vi "getConfiguration.vi"(8 "error in (no error)":errorcluster, 11 "Camera in":refnum<class "Camera.lvclass">) -> (0 "error out":errorcluster, 2 "configuration":T2={"exposure_time_s"=nan, "delay_time_s"=nan, "roi"={"x0"=18446744073709551615, "y0"=18446744073709551615, "x1"=18446744073709551615, "y1"=18446744073709551615}, "timestamp_mode"=65535, "pixelrate"=4294967295, "conversion_factor"=0.0, "trigger_mode"=65535, "acquire_mode"=65535, "acquire_sequence_number"=65535, "metadata_mode"=65535, "noisefilter_mode"=65535, "pixel_format"=0, "binning"={"vert"=0, "horz"=0, "mode"=0}, "auto_exposure"={"region"=0, "min_exposure_s"=0.001, "max_exposure_s"=0.1}} {"conversion_factor" format="%.2g"; "acquire_sequence_number" items=["Undefined"=65535, "OFF"=0, "ON"=1]; "auto_exposure"."region" items=["balanced", "center_based", "corner_based", "full", "custom"]; "binning"."mode" items=["sum", "average"]; "noisefilter_mode" items=["Undefined"=65535, "OFF"=0, "ON"=1]; "exposure_time_s" format="%#_6f"; "timestamp_mode" items=["Undefined"=65535, "OFF"=0, "Binary"=1, "Binary+ASCII"=2, "ASCII"=3]; "acquire_mode" items=["Undefined"=65535, "auto"=0, "external"=1, "external modulate"=2]; "trigger_mode" items=["Undefined"=65535, "auto sequence"=0, "software trigger"=1, "external exposure start & software trigger"=2, "external exposure control"=3, "external synchronized"=4, "fast external exposure control"=5, "external CDS control"=6, "slow external exposure control"=7, "external synchronized HDSDI"=258]; "metadata_mode" items=["Undefined"=65535, "OFF"=0, "ON"=1]}, 3 "Camera out":refnum<class "Camera.lvclass">)   [LabVIEW 2019, in "Camera.lvclass"]
doc: "Gets the current configuration from the camera."
uses:
  Camera.lvclass
  Camera.lvclass/Camera.ctl
  pco.sdk/TimingControl/TimingControl.lvlib
  pco.sdk/ImageSensor/ImageSensor.lvlib
  pco.sdk/RecordingControl/RecordingControl.lvlib
  Controls/binning.ctl
  pco.sdk/GeneralCameraControl/GeneralCameraControl.lvlib
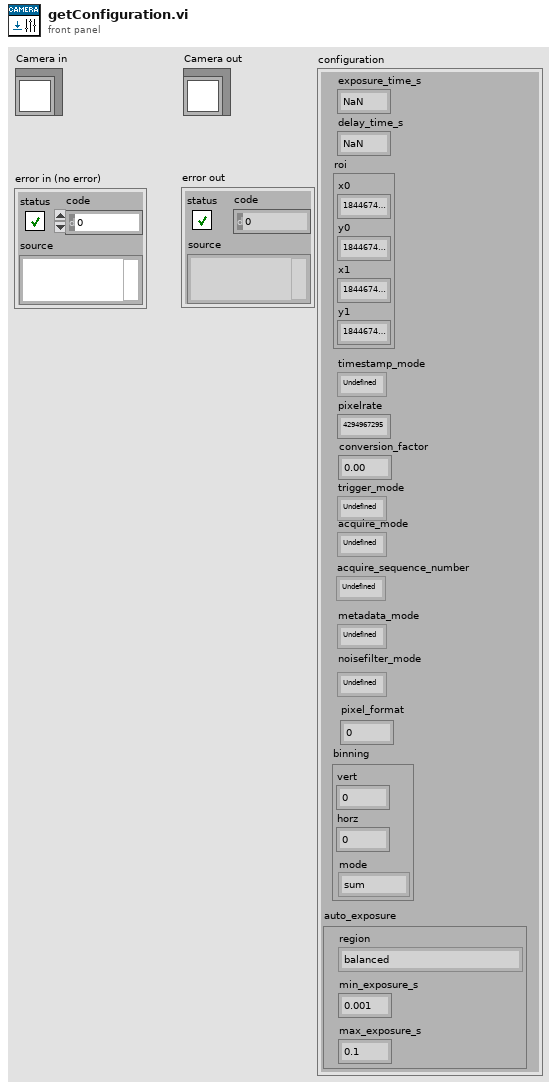
[diagram p1: front panel]
types:
  T1 = typedef "Camera.lvclass/binning.ctl" = cluster{"vert":u16, "horz":u16, "mode":u16}
  T2 = cluster{"exposure_time_s":dbl, "delay_time_s":dbl, "roi":cluster{"x0":u64, "y0":u64, "x1":u64, "y1":u64}, "timestamp_mode":u16, "pixelrate":u32, "conversion_factor":sgl, "trigger_mode":u16, "acquire_mode":u16, "acquire_sequence_number":u32, "metadata_mode":u16, "noisefilter_mode":u16, "pixel_format":u32, "binning":T1, "auto_exposure":cluster{"region":u16, "min_exposure_s":dbl, "max_exposure_s":dbl}}
  T3 = enum16{"SETUP_TYPE_SHUTTERMODE", "SETUP_TYPE_PIXELFORMAT", "SETUP_TYPE_SENSOR_DYNRES"}
  T4 = cluster{"wSensorTypeDESC":u16, "wSensorSubTypeDESC":u16, "wMaxHorzResStdDESC":u16, "wMaxVertResStdDESC":u16, "wMaxHorzResExtDESC":u16, "wMaxVertResExtDESC":u16, "wDynResDESC":u16, "wMaxBinHorzDESC":u16, "wBinHorzSteppingDESC":u16, "wMaxBinVertDESC":u16, "wBinVertSteppingDESC":u16, "wRoiHorStepsDESC":u16, "wRoiVertStepsDESC":u16, "wNumADCsDESC":u16, "wMinSizeHorzDESC":u16, "dwPixelRateDESC":u32[], "wConvFactDESC":u16[], "sCoolingSetpoints":i16[], "wSoftRoiHorStepsDESC":u16, "wSoftRoiVertStepsDESC":u16, "wIRDESC":u16, "wMinSizeVertDESC":u16, "dwMinDelayDESC":u32, "dwMaxDelayDESC":u32, "dwMinDelayStepDESC":u32, "dwMinExposureDESC":u32, "dwMaxExposureDESC":u32, "dwMinExposureStepDESC":u32, "dwMinDelayIRDESC":u32, "dwMaxDelayIRDESC":u32, "dwMinExposureIRDESC":u32, "dwMaxExposureIRDESC":u32, "wTimeTableDESC":u16, "wDoubleImageDESC":u16, "sMinCoolSetDESC":i16, "sMaxCoolSetDESC":i16, "sDefaultCoolSetDESC":i16, "wPowerDownModeDESC":u16, "wOffsetRegulationDESC":u16, "wColorPatternDESC":u16, "wPatternTypeDESC":u16, "wNumCoolingSetpoints":u16, "dwGeneralCapsDESC1":u32, "dwGeneralCapsDESC2":u32, "dwExtSyncFrequency":u32[], "dwGeneralCapsDESC3":u32, "dwGeneralCapsDESC4":u32}
  T5 = cluster{"region":u16, "min_exposure_s":dbl, "max_exposure_s":dbl}
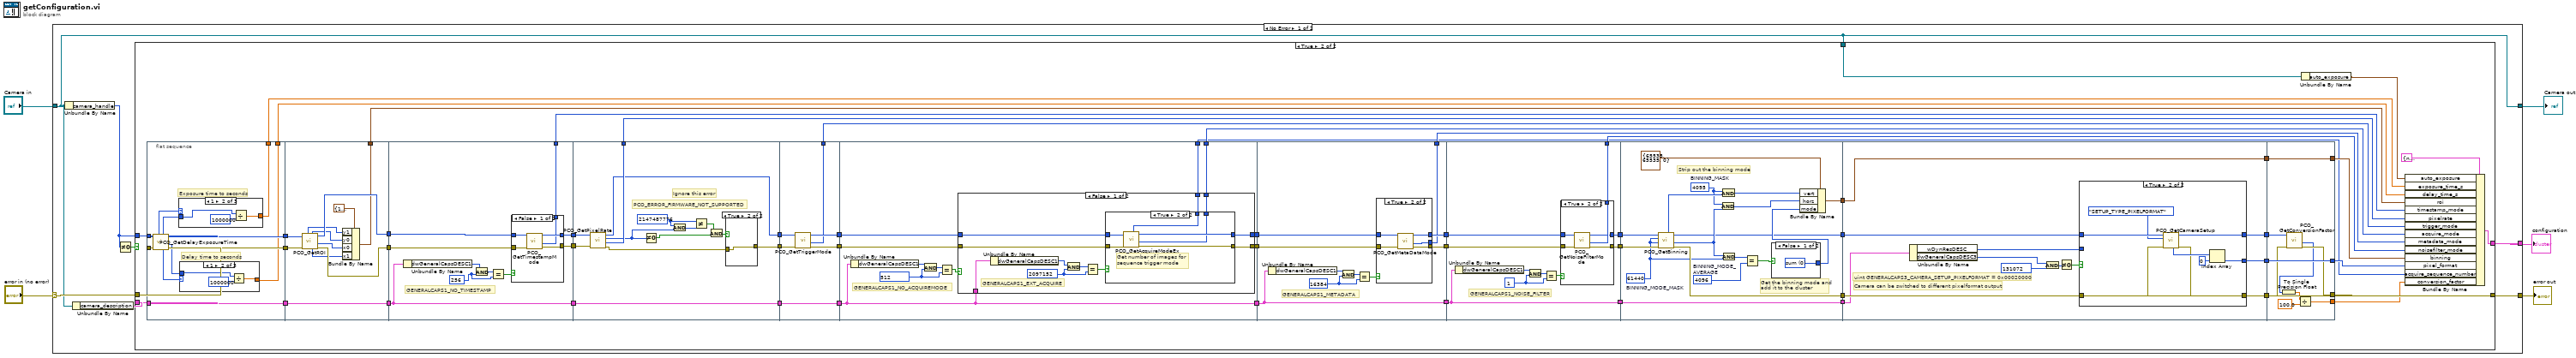
[diagram p0: block diagram]
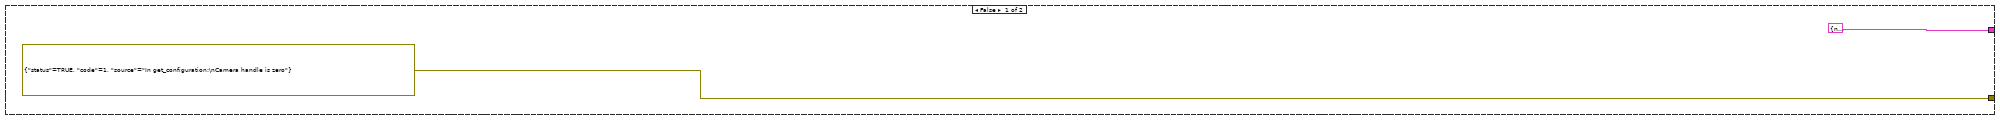
[diagram p2: hidden frame]
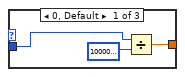
[diagram p3: hidden frame]
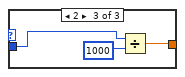
[diagram p4: hidden frame]
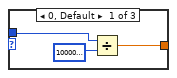
[diagram p5: hidden frame]
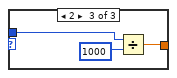
[diagram p6: hidden frame]
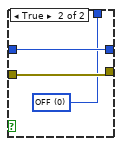
[diagram p7: hidden frame]
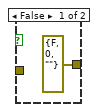
[diagram p8: hidden frame]
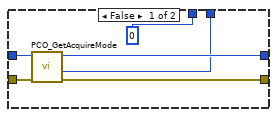
[diagram p9: hidden frame]
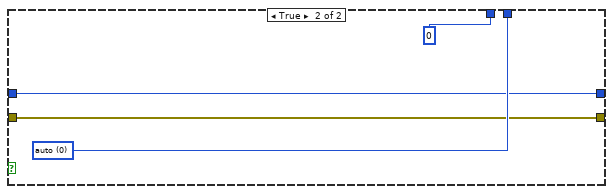
[diagram p10: hidden frame]
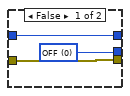
[diagram p11: hidden frame]
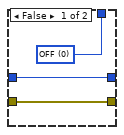
[diagram p12: hidden frame]
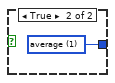
[diagram p13: hidden frame]
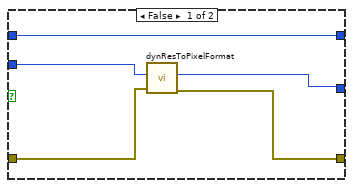
[diagram p14: hidden frame]
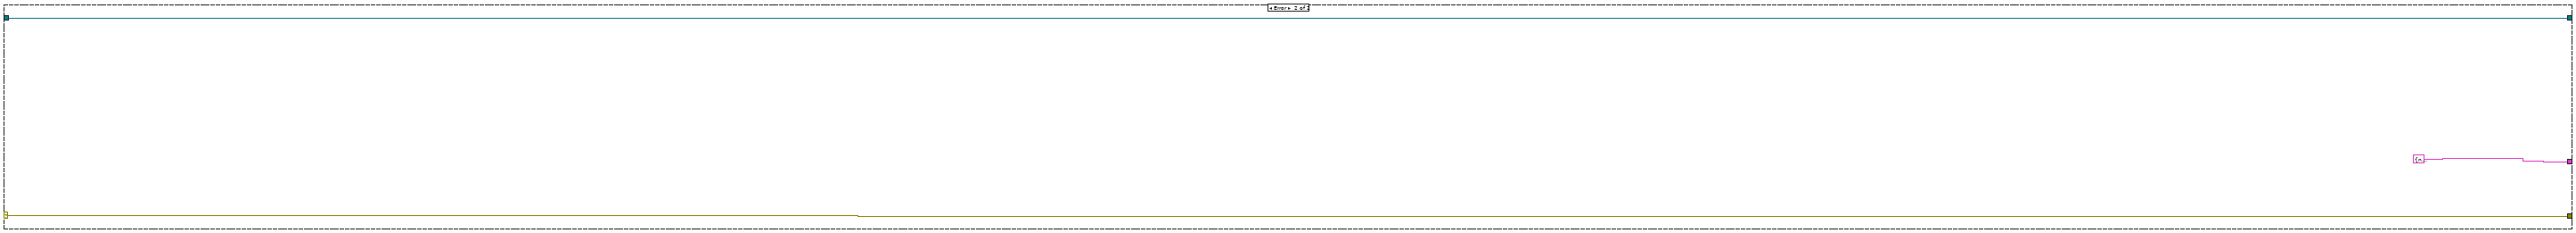
[diagram p15: hidden frame]
diagram:
  n1 = case shown="No Error" "error in (no error)" {
    selector: "error in (no error)" -> [w9 w276]
    tunnel: [w11 w276] -> w4
    tunnel: [w6 w275] -> w2
    tunnel: "Camera in" -> [w6 w275]
    tunnel: [w8 T2 {"exposure_time_s"=nan, "delay_time_s"=nan, "roi"={"x0"=18446744073709551615, "y0"=18446744073709551615, "x1"=18446744073709551615, "y1"=18446744073709551615}, "timestamp_mode"=65535, "pixelrate"=4294967295, "conversion_factor"=0.0, "trigger_mode"=65535, "acquire_mode"=65535, "acquire_sequence_number"=65535, "metadata_mode"=65535, "noisefilter_mode"=65535, "pixel_format"=0, "binning"={"vert"=0, "horz"=0, "mode"=0}, "auto_exposure"={"region"=0, "min_exposure_s"=0.001, "max_exposure_s"=0.1}} ("configuration")] -> w1
    frame No Error {
      n2 = Unbundle By Name(w6) -> ("camera_handle"=w10:u64)
      n3 = Unbundle By Name(w6) -> ("camera_description"=w7:T4)
      n4 = Not Equal To 0?(x=w10) -> (x != 0?=w12:bool)
      n5 = case shown="True" w12 {
        tunnel: [errorcluster {"status"=TRUE, "code"=1, "source"="In get_configuration:\nCamera handle is zero"} ("error constant") w32] -> w11
        tunnel: w10 -> [_ w35]
        tunnel: w9 -> [_ w36]
        tunnel: [T2 {"exposure_time_s"=nan, "delay_time_s"=nan, "roi"={"x0"=18446744073709551615, "y0"=18446744073709551615, "x1"=18446744073709551615, "y1"=18446744073709551615}, "timestamp_mode"=65535, "pixelrate"=4294967295, "conversion_factor"=0.0, "trigger_mode"=65535, "acquire_mode"=65535, "acquire_sequence_number"=65535, "metadata_mode"=65535, "noisefilter_mode"=65535, "pixel_format"=0, "binning"={"vert"=0, "horz"=0, "mode"=0}, "auto_exposure"={"region"=0, "min_exposure_s"=0.001, "max_exposure_s"=0.1}} ("configuration") w22] -> w8
        tunnel: w7 -> [_ w34]
        tunnel: w6 -> [_ w30]
        frame False {
        }
        frame True {
          n6 = flat-sequence {
            tunnel: [w74] -> w67
            tunnel: [w73] -> w66
            tunnel: [w72] -> w55
            tunnel: [w71] -> w54
            tunnel: [w68] -> w48
            tunnel: w36 -> [w70]
            tunnel: w35 -> [w69]
            tunnel: w34 -> [w68]
            tunnel: w67 -> [w106]
            tunnel: w66 -> [w107]
            tunnel: [w104] -> w65
            tunnel: [w103] -> w64
            tunnel: [w97] -> w33
            tunnel: [w98] -> w49
            tunnel: w48 -> [w98]
            tunnel: w65 -> [w116]
            tunnel: w64 -> [w117]
            tunnel: [w115] -> w63
            tunnel: [w114] -> w62
            tunnel: [w113] -> w53
            tunnel: w49 -> [w108]
            tunnel: [w108] -> w44
            tunnel: w63 -> [w138]
            tunnel: w62 -> [w137]
            tunnel: [w127] -> w59
            tunnel: [w126] -> w57
            tunnel: [w136] -> w52
            tunnel: [w135] -> w45
            tunnel: w44 -> [w135]
            tunnel: w59 -> [w146]
            tunnel: [w143] -> w58
            tunnel: w57 -> [w145]
            tunnel: [w144] -> w56
            tunnel: [w142] -> w51
            tunnel: [w141] -> w46
            tunnel: w45 -> [w141]
            tunnel: w58 -> [w157]
            tunnel: w56 -> [w156]
            tunnel: [w153] -> w50
            tunnel: [w155] -> w61
            tunnel: [w154] -> w60
            tunnel: [w148] -> w47
            tunnel: w46 -> [w148]
            tunnel: [w147] -> w21
            tunnel: w61 -> [w187]
            tunnel: w60 -> [w186]
            tunnel: [w190] -> w42
            tunnel: [w189] -> w40
            tunnel: [w188] -> w43
            tunnel: w47 -> [w185]
            tunnel: [w185] -> w38
            tunnel: w42 -> [w207]
            tunnel: [w205] -> w41
            tunnel: w40 -> [w208]
            tunnel: [w204] -> w39
            tunnel: w38 -> [w203]
            tunnel: [w206] -> w37
            tunnel: [w203] -> w24
            tunnel: w41 -> [w237]
            tunnel: w39 -> [w236]
            tunnel: [w224] -> w28
            tunnel: [w235] -> w27
            tunnel: [w222] -> w26
            tunnel: [w221] -> w25
            tunnel: w24 -> [w221]
            tunnel: w28 -> [w251]
            tunnel: w27 -> [w250]
            tunnel: w26 -> [w248]
            tunnel: w25 -> [w244]
            tunnel: [w251] -> w19
            tunnel: [w249] -> w18
            tunnel: [w241] -> w17
            tunnel: [w240] -> w16
            tunnel: [w272] -> w23
            tunnel: [w269] -> w32
            tunnel: [w273] -> w31
            tunnel: w19 -> [w273]
            tunnel: w18 -> [w270]
            tunnel: w17 -> [w272]
            tunnel: w16 -> [w271]
            tunnel: [w265] -> w15
            frame #0 {
              # "Delay time to seconds"
              # "Exposure time to seconds"
              n7 = call "PCO_GetDelayExposureTime.vi"("error in (no error)"=w70, "ph"=w69) -> ("error out"=w73:errorcluster, "dwDelay"=w75:u32, "ph out"=w74:u64, "wTimeBaseDelay"=w78:u16, "dwExposure"=w76:u32, "wTimeBaseExposure"=w77:u16)  [unwired: 3 in, 1 out]
              n8 = case shown="1" w77 {
                tunnel: w76 -> [w80 w83 w86]
                tunnel: [w79 w82 w85] -> w72
                frame 0, Default {
                  n9 = Divide(x=w80, y=u32 1000000000) -> (x/y=w79:dbl)
                }
                frame 1 {
                  n10 = Divide(x=w83, y=u32 1000000) -> (x/y=w82:dbl)
                }
                frame 2 {
                  n11 = Divide(x=w86, y=u32 1000) -> (x/y=w85:dbl)
                }
              }
              n12 = case shown="1" w78 {
                tunnel: w75 -> [w90 w92 w95]
                tunnel: [w88 w91 w94] -> w71
                frame 0, Default {
                  n13 = Divide(x=w90, y=u32 1000000000) -> (x/y=w88:dbl)
                }
                frame 1 {
                  n14 = Divide(x=w92, y=u32 1000000) -> (x/y=w91:dbl)
                }
                frame 2 {
                  n15 = Divide(x=w95, y=u32 1000) -> (x/y=w94:dbl)
                }
              }
            }
            frame #1 {
              n16 = call "PCO_GetROI.vi"("error in (no error)"=w107, "ph"=w106) -> ("error out"=w104:errorcluster, "wRoiX0"=w102:u16, "ph out"=w103:u64, "wRoiX1"=w101:u16, "wRoiY0"=w100:u16, "wRoiY1"=w99:u16)  [unwired: 3 in, 1 out]
              n17 = Bundle By Name(cluster=cluster{"x0":u64, "y0":u64, "x1":u64, "y1":u64} {"x0"=18446744073709551615, "y0"=18446744073709551615, "x1"=18446744073709551615, "y1"=18446744073709551615}, "y1"=w99, "y0"=w100, "x0"=w102, "x1"=w101) -> (w97:cluster{"x0":u64, "y0":u64, "x1":u64, "y1":u64})
            }
            frame #2 {
              w110 = u32 256 ("y")
              # "GENERALCAPS1_NO_TIMESTAMP"
              n18 = Unbundle By Name(w108) -> ("dwGeneralCapsDESC1"=w111:u32)
              n19 = And(x=w111, y=w110) -> (x .and. y?=w112:u32)
              n20 = Equal?(x=w112, y=w110) -> (x = y?=w109:bool)
              n21 = case shown="False" w109 {
                tunnel: w117 -> [w122 w125]
                tunnel: w116 -> [w121 w124]
                tunnel: [w120 w124] -> w115
                tunnel: [w119 w125] -> w114
                tunnel: [w118 w123] -> w113
                frame False {
                  n22 = call "PCO_GetTimestampMode.vi"("error in (no error)"=w121, "ph"=w122) -> ("error out"=w120:errorcluster, "wTimeStampMode"=w118:u16, "ph out"=w119:u64)  [unwired: 6 in, 1 out]
                }
                frame True {
                  w123 = u16 0 items=["OFF", "Binary", "Binary+ASCII", "ASCII"] ("wTimeStampMode")
                }
              }
            }
            frame #3 {
              w132 = u32 2147487776
              # "Ignore this error"
              # "PCO_ERROR_FIRMWARE_NOT_SUPPORTED"
              n23 = call "PCO_GetPixelRate.vi"("error in (no error)"=w138, "ph"=w137) -> ("error out"=w128:errorcluster, "dwPixelRate"=w136:u32, "ErrorMessage"=w134:i32, "ph out"=w126:u64)  [unwired: 6 in]
              n24 = Not Equal To 0?(x=w134) -> (x != 0?=w130:bool)
              n25 = And(x=w132, y=w134) -> (x .and. y?=w133:u32)
              n26 = Not Equal?(x=w132, y=w133) -> (x != y?=w131:bool)
              n27 = And(x=w131, y=w130) -> (x .and. y?=w129:bool)
              n28 = case shown="True" w129 {
                tunnel: w128 -> [_ w140]
                tunnel: [errorcluster {"status"=FALSE, "code"=0, "source"=""} ("error out") w140] -> w127
                frame False {
                }
                frame True {
                }
              }
            }
            frame #4 {
              n29 = call "PCO_GetTriggerMode.vi"("error in (no error)"=w146, "ph"=w145) -> ("error out"=w143:errorcluster, "wTriggerMode"=w142:u16, "ph out"=w144:u64)  [unwired: 6 in, 1 out]
            }
            frame #5 {
              w150 = u32 512 ("y")
              # "GENERALCAPS1_NO_ACQUIREMODE"
              n30 = Unbundle By Name(w148) -> ("dwGeneralCapsDESC1"=w152:u32)
              n31 = And(x=w152, y=w150) -> (x .and. y?=w151:u32)
              n32 = Equal?(x=w151, y=w150) -> (x = y?=w149:bool)
              n33 = case shown="False" w149 {
                tunnel: w157 -> [w168 w182]
                tunnel: w156 -> [w167 w183]
                tunnel: [w166 w183] -> w155
                tunnel: [w165 w182] -> w154
                tunnel: [w164 w184] -> w153
                tunnel: w148 -> [w163 _]
                tunnel: [w158 u32 0 ("dwNumberImages")] -> w147
                frame False {
                  w160 = u32 2097152 ("y")
                  # "GENERALCAPS1_EXT_ACQUIRE"
                  n34 = Unbundle By Name(w163) -> ("dwGeneralCapsDESC1"=w162:u32)
                  n35 = And(x=w162, y=w160) -> (x .and. y?=w161:u32)
                  n36 = Equal?(x=w161, y=w160) -> (x = y?=w159:bool)
                  n37 = case shown="True" w159 {
                    tunnel: w168 -> [w174 w180]
                    tunnel: w167 -> [w173 w179]
                    tunnel: [w172 w177] -> w166
                    tunnel: [w171 w178] -> w165
                    tunnel: [w170 w176] -> w164
                    tunnel: [u32 0 ("dwNumberImages") w175] -> w158
                    frame False {
                      n38 = call "PCO_GetAcquireMode.vi"("error in (no error)"=w174, "ph"=w173) -> ("error out"=w171:errorcluster, "wAcquMode"=w170:u16, "ph out"=w172:u64)  [unwired: 6 in, 1 out]
                    }
                    frame True {
                      # "Get number of images for sequence trigger mode"
                      n39 = call "PCO_GetAcquireModeEx.vi"("error in (no error)"=w180, "ph"=w179) -> ("error out"=w178:errorcluster, "wAcquMode"=w176:u16, "ph out"=w177:u64, "dwNumberImages"=w175:u32)  [unwired: 5 in, 1 out]
                    }
                  }
                }
                frame True {
                  w184 = u16 0 items=["auto", "external", "external modulate"] ("wAcquMode")
                }
              }
            }
            frame #6 {
              w192 = u32 16384 ("y")
              # "GENERALCAPS1_METADATA"
              n40 = Unbundle By Name(w185) -> ("dwGeneralCapsDESC1"=w194:u32)
              n41 = And(x=w194, y=w192) -> (x .and. y?=w193:u32)
              n42 = Equal?(x=w193, y=w192) -> (x = y?=w191:bool)
              n43 = case shown="True" w191 {
                tunnel: w187 -> [w197 w202]
                tunnel: w186 -> [w195 w201]
                tunnel: [w197 w200] -> w190
                tunnel: [w195 w199] -> w189
                tunnel: [w196 w198] -> w188
                frame False {
                  w196 = u16 0 items=["OFF", "ON"] ("wMetaDataMode")
                }
                frame True {
                  n44 = call "PCO_GetMetaDataMode.vi"("error in (no error)"=w201, "ph"=w202) -> ("error out"=w199:errorcluster, "wMetaDataMode"=w198:u16, "ph out"=w200:u64)  [unwired: 4 in, 3 out]
                }
              }
            }
            frame #7 {
              w210 = u32 1 ("y")
              # "GENERALCAPS1_NOISE_FILTER"
              n45 = Unbundle By Name(w203) -> ("dwGeneralCapsDESC1"=w212:u32)
              n46 = And(x=w212, y=w210) -> (x .and. y?=w211:u32)
              n47 = Equal?(x=w211, y=w210) -> (x = y?=w209:bool)
              n48 = case shown="True" w209 {
                tunnel: w208 -> [w213 w220]
                tunnel: w207 -> [w214 w219]
                tunnel: [w215 w218] -> w206
                tunnel: [w214 w217] -> w205
                tunnel: [w213 w216] -> w204
                frame False {
                  w215 = u16 0 items=["OFF", "ON"] ("noisefilter_mode")
                }
                frame True {
                  n49 = call "PCO_GetNoiseFilterMode.vi"("error in (no error)"=w220, "ph"=w219) -> ("error out"=w216:errorcluster, "wNoiseFilterMode"=w218:u16, "ph out"=w217:u64)  [unwired: 6 in, 1 out]
                }
              }
            }
            frame #8 {
              w225 = u16 61440  # BINNING_MODE_MASK
              w228 = u16 4096  # BINNING_MODE_AVERAGE
              w232 = u16 4095  # BINNING_MASK
              # "Get the binning mode and add it to the cluster"
              # "Strip out the binning mode"
              n50 = call "PCO_GetBinning.vi"("error in (no error)"=w236, "wBinVertIn"=w225, "wBinHorzIn"=w225, "ph"=w237) -> ("error out"=w235:errorcluster, "wBinHorz"=w230:u16, "ph out"=w222:u64, "wBinVert"=w234:u16)  [unwired: 3 in, 1 out]
              n51 = And(x=w232, y=w230) -> (x .and. y?=w231:u16)
              n52 = And(x=w232, y=w234) -> (x .and. y?=w233:u16)
              n53 = And(x=w230, y=w225) -> (x .and. y?=w229:u16)
              n54 = Equal?(x=w229, y=w228) -> (x = y?=w227:bool)
              n55 = case shown="False" w227 {
                tunnel: [w238 w239] -> w226
                frame False {
                  w238 = u16 0 items=["sum", "average"] ("BinningMode")
                }
                frame True {
                  w239 = u16 1 items=["sum", "average"] ("BinningMode")
                }
              }
              n56 = Bundle By Name(cluster=T1 {"vert"=65535, "horz"=65535, "mode"=0} ("binning"), "vert"=w233, "horz"=w231, "mode"=w226) -> (w224:T1)
            }
            frame #9 {
              # "Camera can be switched to different pixelformat output"
              # "uint GENERALCAPS3_CAMERA_SETUP_PIXELFORMAT = 0x00020000"
              n57 = Unbundle By Name(w244) -> ("wDynResDESC"=w242:u16, "dwGeneralCapsDESC3"=w247:u32)
              n58 = And(x=w247, y=u32 131072) -> (x .and. y?=w246:u32)
              n59 = Not Equal To 0?(x=w246) -> (x != 0?=w243:bool)
              n60 = case shown="True" w243 {
                tunnel: w250 -> [w254 w262]
                tunnel: [w253 w261] -> w249
                tunnel: w248 -> [w252 w260]
                tunnel: [w255 w259] -> w241
                tunnel: w242 -> [w256 _]
                tunnel: [w252 w257] -> w240
                frame False {
                  n61 = call "dynResToPixelFormat.vi"("error in (no error)"=w254, "dyn_res"=w256) -> ("error out"=w253:errorcluster, "PixelFormat"=w255:u32)  [unwired: 8 in]
                }
                frame True {
                  n62 = call "PCO_GetCameraSetup.vi"("error in (no error)"=w262, "wTypeIn"=T3."SETUP_TYPE_PIXELFORMAT", "ph"=w260) -> ("error out"=w261:errorcluster, "ph out"=w257:u64, "dwSetup"=w264:u32[])  [unwired: 4 in, 2 out]
                  n63 = Index Array(array=w264, index=0) -> (element=w259:u32)
                }
              }
            }
            frame #10 {
              n64 = call "PCO_GetConversionFactor.vi"("error in (no error)"=w270, "ph"=w271) -> ("error out"=w269:errorcluster, "wConvFact"=w268:u16)  [unwired: 6 in, 2 out]
              n65 = To Single Precision Float(number=w268) -> (single precision float=w267:sgl)
              n66 = Divide(x=w267, y=sgl 100.0) -> (x/y=w265:sgl)
            }
          }
          n67 = Unbundle By Name(w30) -> ("auto_exposure"=w29:T5)
          n68 = Bundle By Name(cluster=T2 {"exposure_time_s"=nan, "delay_time_s"=nan, "roi"={"x0"=18446744073709551615, "y0"=18446744073709551615, "x1"=18446744073709551615, "y1"=18446744073709551615}, "timestamp_mode"=65535, "pixelrate"=4294967295, "conversion_factor"=0.0, "trigger_mode"=65535, "acquire_mode"=65535, "acquire_sequence_number"=65535, "metadata_mode"=65535, "noisefilter_mode"=65535, "pixel_format"=0, "binning"={"vert"=0, "horz"=0, "mode"=0}, "auto_exposure"={"region"=0, "min_exposure_s"=0.001, "max_exposure_s"=0.1}} ("configuration"), "auto_exposure"=w29, "exposure_time_s"=w55, "delay_time_s"=w54, "roi"=w33, "timestamp_mode"=w53, "pixelrate"=w52, "trigger_mode"=w51, "acquire_mode"=w50, "metadata_mode"=w43, "noisefilter_mode"=w37, "binning"=w31, "pixel_format"=w23, "acquire_sequence_number"=w21, "conversion_factor"=w15) -> (w22:T2)
        }
      }
    }
    frame Error {
    }
  }
  "error out" <- w4
  "Camera out" <- w2
  "configuration" <- w1
